vi "Force To Voltage.vi"(8 "error in (no error)":errorcluster, 9 "Turbo Valve Settings":T1={"Bias"=32768, "Minimum Voltage"=0.0, "Maximum Voltage"=4.096, "Off Value"=0.0} {"Off Value" format="%.3f"; "Maximum Voltage" format="%.3f"; "Minimum Voltage" format="%.3f"; "Bias" step=1}, 10 "Percentage":dbl, 11 "Force To Pressure Servo Valve Voltage in":refnum<class "Percentage To Turbo Valve Voltage.lvclass">) -> (0 "error out":errorcluster, 2 "Voltage":dbl[unit], 3 "Force To Pressure Servo Valve Voltage out":refnum<class "Percentage To Turbo Valve Voltage.lvclass">)   [LabVIEW 2015, in "Percentage To Turbo Valve Voltage.lvclass"]
uses:
  Percentage To Turbo Valve Voltage.lvclass
  Typedefs/Turbo Valve Settings.ctl
  Typedefs/FAMT Typedefs.lvlib
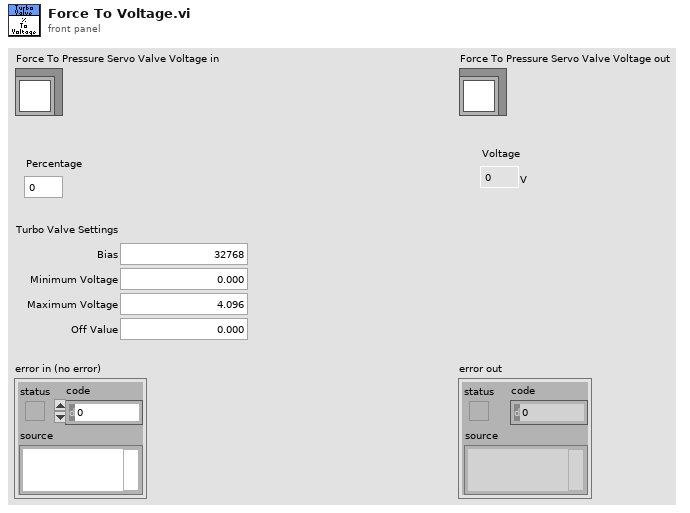
[diagram p1: front panel]
types:
  T1 = typedef "FAMT Typedefs.lvlib/Turbo Valve Settings.ctl" = cluster{"Bias":u16, "Minimum Voltage":dbl, "Maximum Voltage":dbl, "Off Value":dbl}
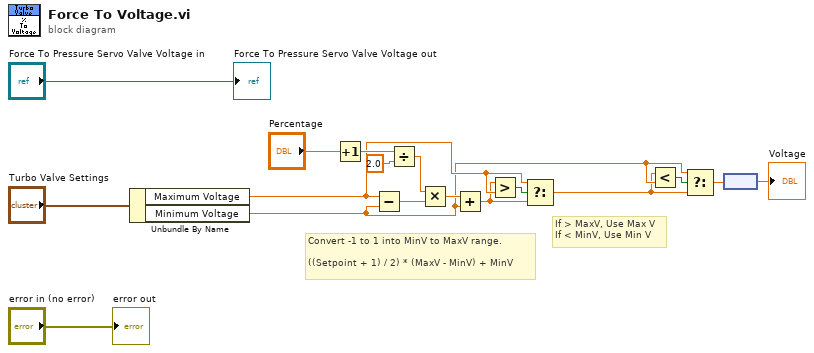
[diagram p0: block diagram]
diagram:
  # "If > MaxV, Use Max V\nIf < MinV, Use Min V"
  # "Convert -1 to 1 into MinV to MaxV range.\n\n((Setpoint + 1) / 2) * (MaxV - MinV) + MinV"
  n1 = Unbundle By Name("Turbo Valve Settings") -> ("Maximum Voltage"=w8:dbl, "Minimum Voltage"=w5:dbl)
  n2 = Increment(x="Percentage") -> (x+1=w14:dbl)
  n3 = Subtract(x=w8, y=w5) -> (x-y=w11:dbl)
  n4 = Divide(x=w14, y=2.0) -> (x/y=w12:dbl)
  n5 = Multiply(x=w12, y=w11) -> (x*y=w10:dbl)
  n6 = Add(x=w10, y=w5) -> (x+y=w7:dbl)
  n7 = Greater?(x=w7, y=w8) -> (0:w9:bool)
  n8 = Select(t=w8, s=w9, f=w7) -> (s? t:f=w4:dbl)
  n9 = Less?(x=w4, y=w5) -> (x < y?=w6:bool)
  n10 = Select(t=w5, s=w6, f=w4) -> (s? t:f=w1:dbl)
  n11 = node(w1) -> (→"Voltage":dbl[unit])
  "error out" <- "error in (no error)"
  "Force To Pressure Servo Valve Voltage out" <- "Force To Pressure Servo Valve Voltage in"
